vi "Close.vi"(8 "error in":errorcluster, 11 "Cell View Alternating Back Color in":refnum<class "Cell View Alternating Back Color.lvclass">) -> (0 "error out":errorcluster, 3 "Cell View Alternating Back Color out":refnum<class "Cell View Alternating Back Color.lvclass">)   [LabVIEW 2024, in "SourceGrid.lvlib" / "Cell View Alternating Back Color.lvclass"]
uses:
  Cell View Alternating Back Color.lvclass
  Cell View Alternating Back Color.lvclass/Cell View Alternating Back Color.ctl
  Cell View/Cell View.lvclass
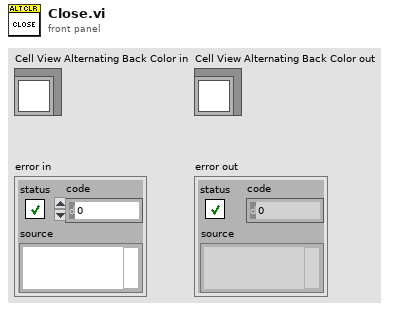
[diagram p1: front panel]
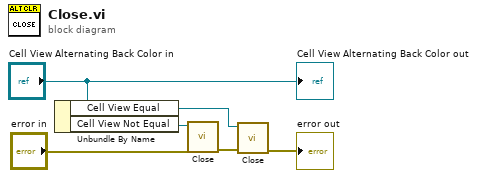
[diagram p0: block diagram]
diagram:
  n1 = Unbundle By Name("Cell View Alternating Back Color in") -> ("Cell View Equal"=w2:refnum<class "Cell View.lvclass">, "Cell View Not Equal"=w4:refnum<class "Cell View.lvclass">)
  n2 = call-dynamic "Close.vi"("error in"="error in", "Cell View in"=w4) -> ("error out"=w3:errorcluster)  [unwired: 8 in, 1 out]
  n3 = call-dynamic "Close.vi"("error in"=w3, "Cell View in"=w2) -> ("error out"=→"error out":errorcluster)  [unwired: 8 in, 1 out]
  "Cell View Alternating Back Color out" <- "Cell View Alternating Back Color in"
